vi "Dash Read.vi"(0 "Auto Options":T5={"Starting Position"=enum."Left L1 ", "First Score Pos"=enum."7", "Second Score Pos"=enum."5"}, 2 "PID gains A":T1={"proportional gain (Kc)"=0.039, "integral time (Ti, min)"=0.0, "derivative time (Td, min)"=0.0018000000000000004} {"derivative time (Td, min)" format="%.4f"; "integral time (Ti, min)" format="%.4f"; "proportional gain (Kc)" format="%.4f"}, 3 "PID gains B":T1={"proportional gain (Kc)"=0.027999999999999997, "integral time (Ti, min)"=0.0, "derivative time (Td, min)"=0.0018000000000000004} {"derivative time (Td, min)" format="%.4f"; "integral time (Ti, min)" format="%.4f"; "proportional gain (Kc)" format="%.4f"}) -> (12 "Competion":string, 14 "Replay Number":dbl, 15 "Match Number":dbl, 16 "Match Type":string, 17 "output cluster":T2, 18 "Pressure":dbl, 19 "AutoValid?":bool)   [LabVIEW 2018]
uses:
  Subsystems/Drive/MotionProfile/StartingPosition.ctl
  Subsystems/Drive/MotionProfile/Path_Decider.ctl
  <vilib>/Rock Robotics/Network Tables/NT Read Boolean.vi
  <vilib>/Rock Robotics/Network Tables/NT Write Variant.vi
  <vilib>/Rock Robotics/Network Tables/NT Read Number.vi
  <vilib>/Rock Robotics/Network Tables/NT Read String.vi
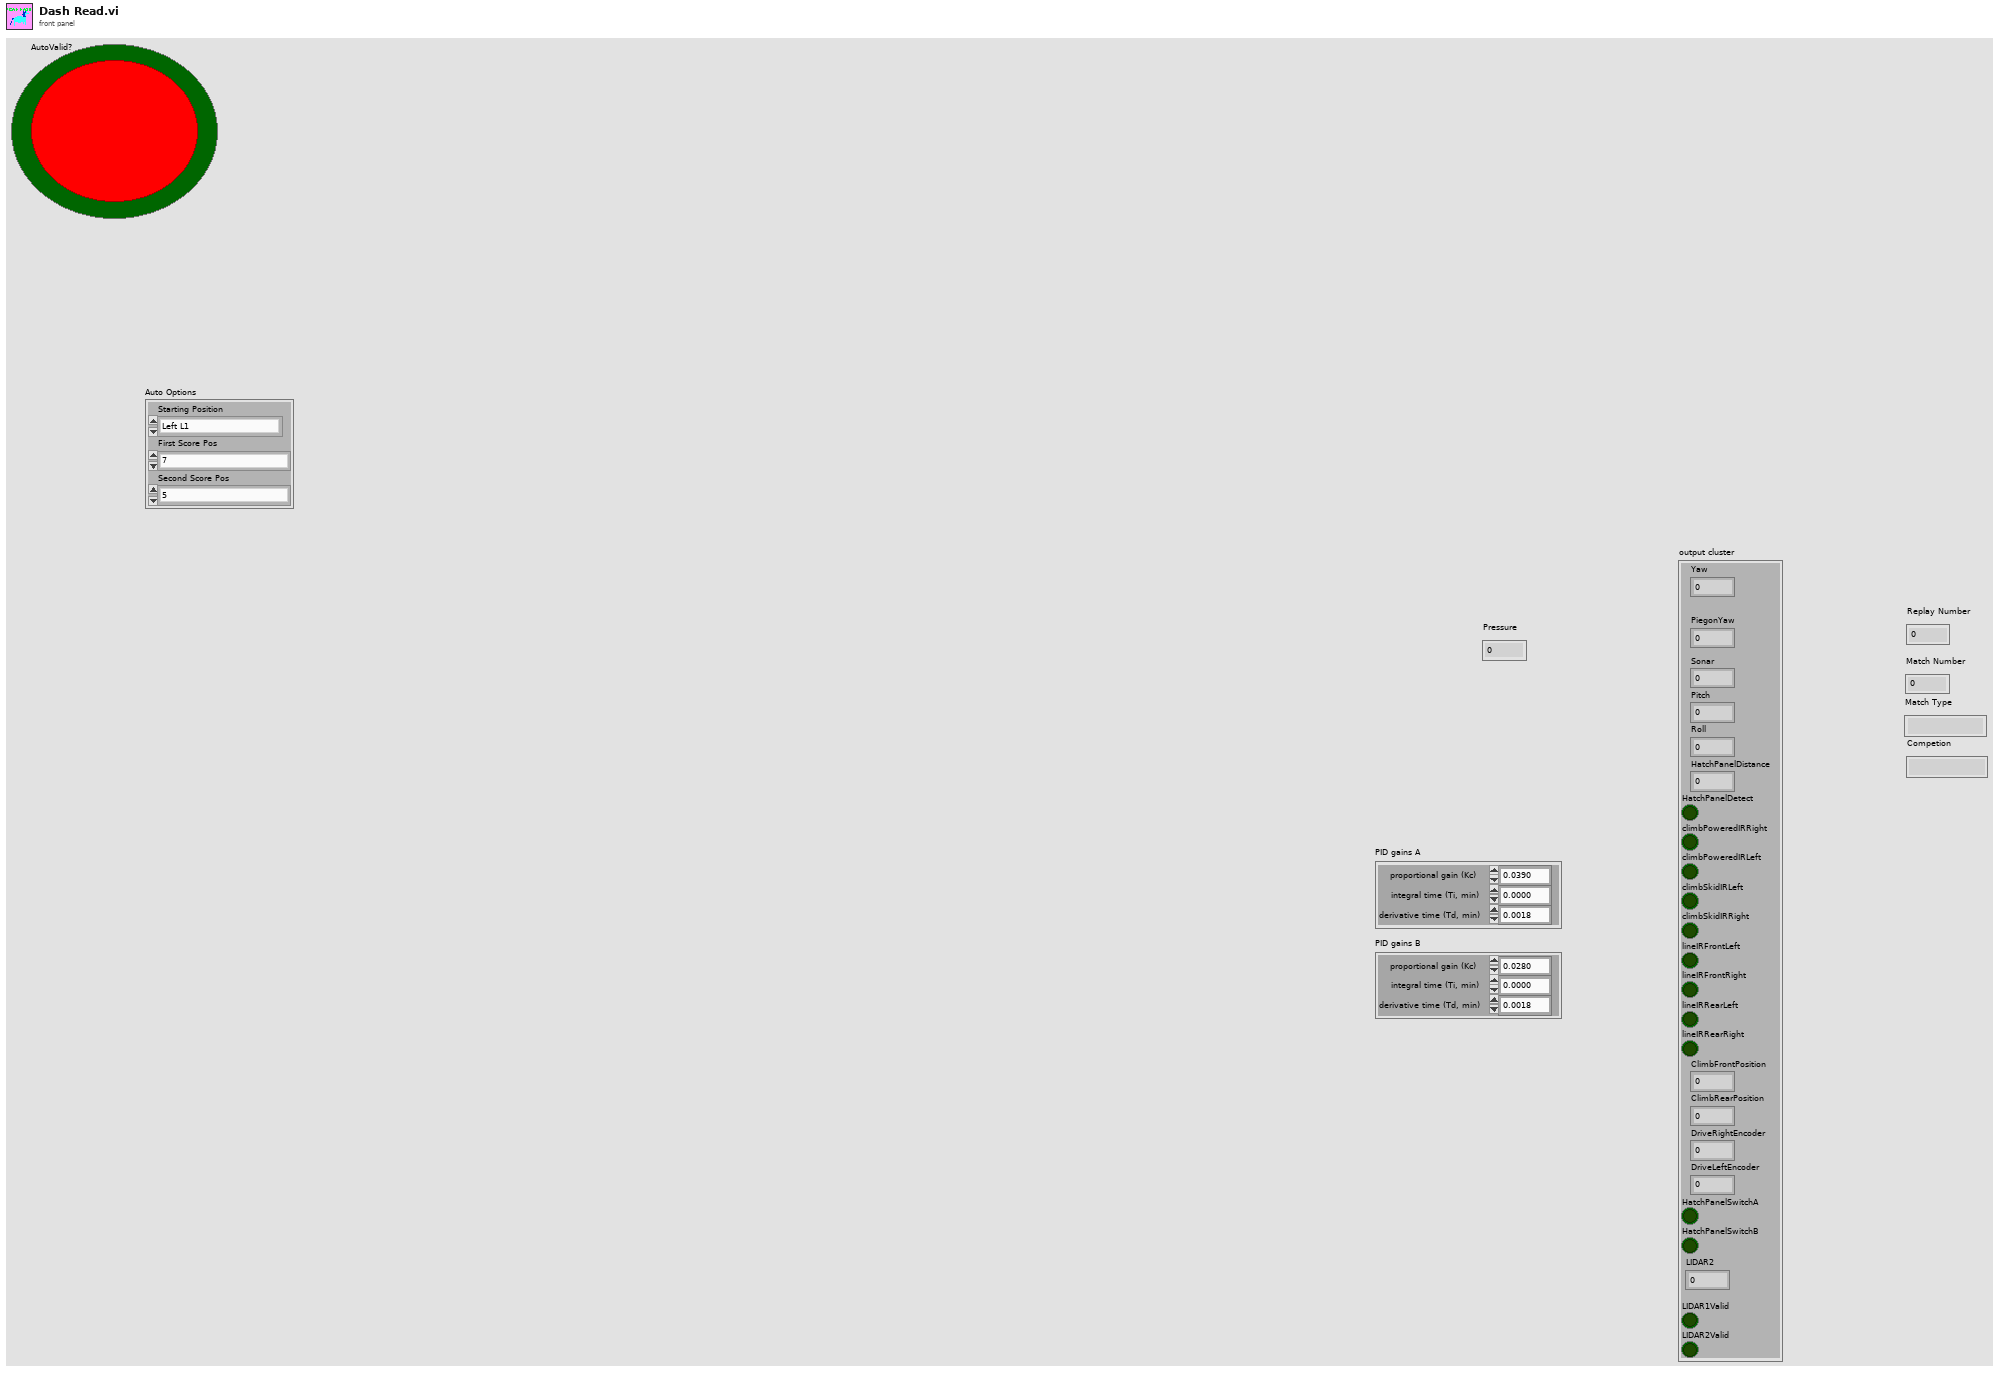
[diagram p1: front panel]
types:
  T1 = cluster{"proportional gain (Kc)":dbl, "integral time (Ti, min)":dbl, "derivative time (Td, min)":dbl}
  T2 = cluster{"Yaw":dbl, "Sonar":dbl, "Pitch":dbl, "Roll":dbl, "HatchPanelDistance":dbl, "HatchPanelDetect":bool, "climbPoweredIRRight":bool, "climbPoweredIRLeft":bool, "climbSkidIRLeft":bool, "climbSkidIRRight":bool, "lineIRFrontLeft":bool, "lineIRFrontRight":bool, "lineIRRearLeft":bool, "lineIRRearRight":bool, "ClimbFrontPosition":dbl, "ClimbRearPosition":dbl, "DriveRightEncoder":dbl, "DriveLeftEncoder":dbl, "HatchPanelSwitchA":bool, "HatchPanelSwitchB":bool, "LIDAR2":dbl, "PiegonYaw":dbl, "LIDAR2Valid":bool, "LIDAR1Valid":bool}
  T3 = typedef "StartingPosition.ctl" = enum16{"Left L1 ", "Middle L1", "Right L1", "Left L2", "Right L2", "Don't Move"}
  T4 = typedef "Path_Decider.ctl" = enum16{"1", "2", "3", "4", "5", "6", "7", "8", "Left_Rocket_Front", "Left_Rocket_Rear", "Right_Rocket_Front", "Right_Rocket_Rear"}
  T5 = cluster{"Starting Position":T3, "First Score Pos":T4, "Second Score Pos":T4}
  T6 = cluster{"Yaw":dbl, "Sonar":dbl, "Pitch":dbl, "Roll":dbl, "HatchPanelDistance":dbl, "HatchPanelDetect":bool, "climbPoweredIRRight":bool, "climbPoweredIRLeft":bool, "climbSkidIRLeft":bool, "climbSkidIRRight":bool, "lineIRFrontLeft":bool, "lineIRFrontRight":bool, "lineIRRearLeft":bool, "lineIRRearRight":bool, "ClimbFrontPosition":dbl, "ClimbRearPosition":dbl, "DriveRightEncoder":dbl, "DriveLeftEncoder":dbl, "HatchPanelSwitchA":bool, "HatchPanelSwitchB":bool, "LIDAR2":dbl, "PigeonYaw":dbl, "LIDAR1Valid":bool, "LIDAR2Valid":bool}
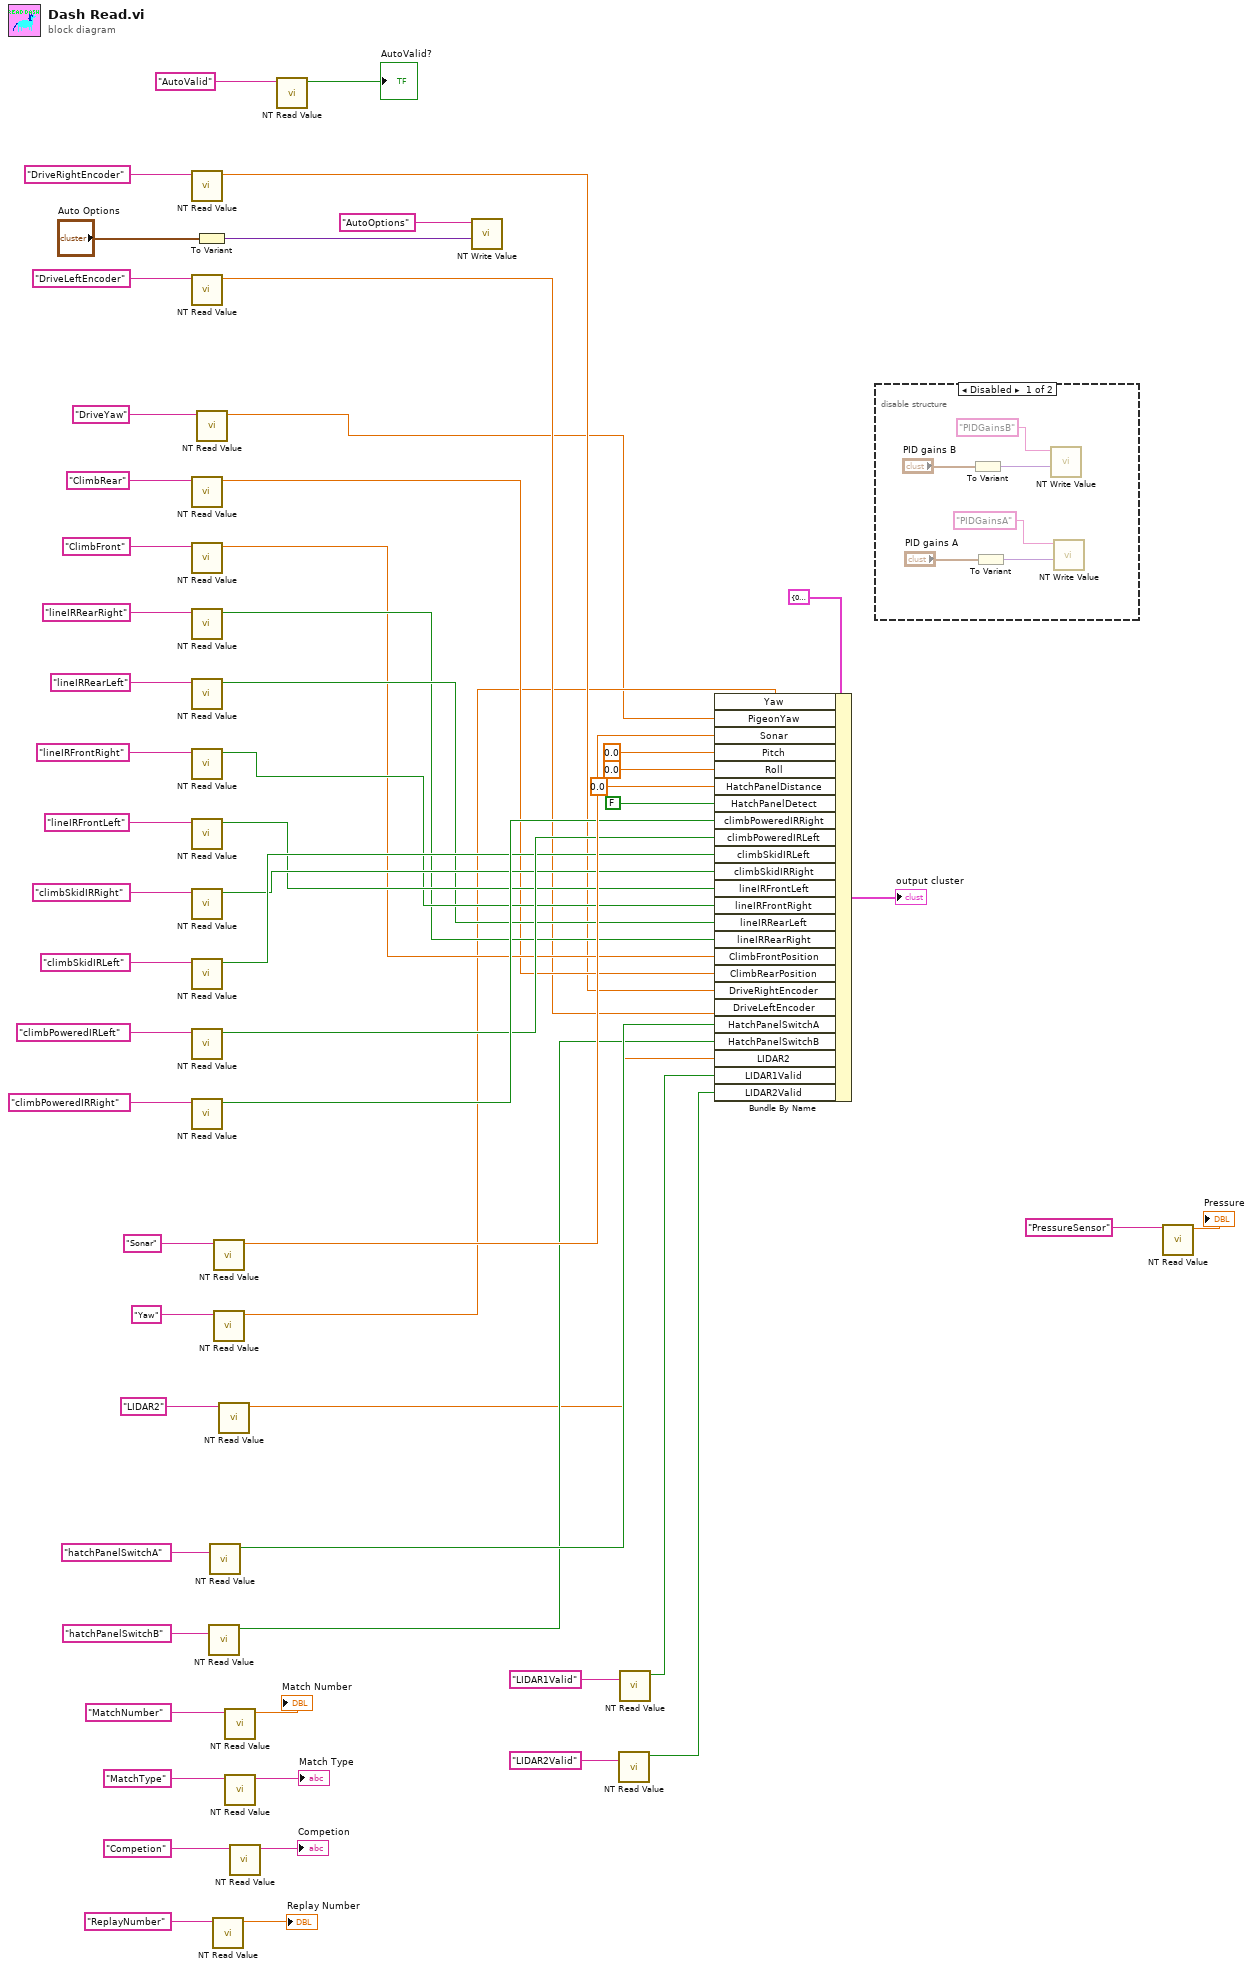
[diagram p0: block diagram]
diagram:
  n1 = call-poly <vilib>:"NT Read Value.vi"("Name"="DriveRightEncoder") -> ("Numeric"=w30:dbl)  [unwired: 9 in, 1 out]
  n2 = call-poly <vilib>:"NT Read Value.vi"("Name"="DriveLeftEncoder") -> ("Numeric"=w29:dbl)  [unwired: 9 in, 1 out]
  n3 = call-poly <vilib>:"NT Read Value.vi"("Name"="ClimbRear") -> ("Numeric"=w31:dbl)  [unwired: 9 in, 1 out]
  n4 = call-poly <vilib>:"NT Read Value.vi"("Name"="ClimbFront") -> ("Numeric"=w32:dbl)  [unwired: 9 in, 1 out]
  n5 = call-poly <vilib>:"NT Read Value.vi"("Name"="lineIRRearRight") -> ("Boolean"=w33:bool)  [unwired: 9 in, 1 out]
  n6 = call-poly <vilib>:"NT Read Value.vi"("Name"="lineIRRearLeft") -> ("Boolean"=w34:bool)  [unwired: 9 in, 1 out]
  n7 = call-poly <vilib>:"NT Read Value.vi"("Name"="lineIRFrontRight") -> ("Boolean"=w35:bool)  [unwired: 9 in, 1 out]
  n8 = call-poly <vilib>:"NT Read Value.vi"("Name"="lineIRFrontLeft") -> ("Boolean"=w36:bool)  [unwired: 9 in, 1 out]
  n9 = call-poly <vilib>:"NT Read Value.vi"("Name"="climbSkidIRRight") -> ("Boolean"=w37:bool)  [unwired: 9 in, 1 out]
  n10 = call-poly <vilib>:"NT Read Value.vi"("Name"="climbSkidIRLeft") -> ("Boolean"=w38:bool)  [unwired: 9 in, 1 out]
  n11 = call-poly <vilib>:"NT Read Value.vi"("Name"="climbPoweredIRLeft") -> ("Boolean"=w39:bool)  [unwired: 9 in, 1 out]
  n12 = call-poly <vilib>:"NT Read Value.vi"("Name"="climbPoweredIRRight") -> ("Boolean"=w40:bool)  [unwired: 9 in, 1 out]
  n13 = To Variant(anything="Auto Options") -> (Variant=w51:variant)
  n14 = call-poly <vilib>:"NT Read Value.vi"("Name"="DriveYaw") -> ("Numeric"=w7:dbl)  [unwired: 9 in, 1 out]
  n15 = call-poly <vilib>:"NT Read Value.vi"("Name"="hatchPanelSwitchB") -> ("Boolean"=w25:bool)  [unwired: 9 in, 1 out]
  n16 = call-poly <vilib>:"NT Read Value.vi"("Name"="hatchPanelSwitchA") -> ("Boolean"=w26:bool)  [unwired: 9 in, 1 out]
  n17 = call-poly <vilib>:"NT Read Value.vi"("Name"="ReplayNumber") -> ("Numeric"=→"Replay Number":dbl)  [unwired: 9 in, 1 out]
  n18 = call-poly <vilib>:"NT Read Value.vi"("Name"="Sonar") -> ("Numeric"=w41:dbl)  [unwired: 9 in, 1 out]
  n19 = call-poly <vilib>:"NT Read Value.vi"("Name"="Yaw") -> ("Numeric"=w13:dbl)  [unwired: 9 in, 1 out]
  n20 = call-poly <vilib>:"NT Read Value.vi"("Name"="LIDAR2") -> ("Numeric"=w8:dbl)  [unwired: 9 in, 1 out]
  n21 = call-poly <vilib>:"NT Read Value.vi"("Name"="MatchNumber") -> ("Numeric"=→"Match Number":dbl)  [unwired: 9 in, 1 out]
  n22 = call-poly <vilib>:"NT Read Value.vi"("Name"="MatchType") -> ("String"=→"Match Type":string)  [unwired: 9 in, 1 out]
  n23 = call-poly <vilib>:"NT Read Value.vi"("Name"="Competion") -> ("String"=→"Competion":string)  [unwired: 9 in, 1 out]
  n24 = call-poly <vilib>:"NT Read Value.vi"("Name"="AutoValid") -> ("Boolean"=→"AutoValid?":bool)  [unwired: 9 in, 1 out]
  n25 = call-poly <vilib>:"NT Write Value.vi"("Variant"=w51, "Name"="AutoOptions") -> ()  [unwired: 9 in, 1 out]
  n26 = call-poly <vilib>:"NT Read Value.vi"("Name"="LIDAR2Valid") -> ("Boolean"=w3:bool)  [unwired: 9 in, 1 out]
  n27 = call-poly <vilib>:"NT Read Value.vi"("Name"="LIDAR1Valid") -> ("Boolean"=w4:bool)  [unwired: 9 in, 1 out]
  n28 = Bundle By Name(cluster=T6 {"Yaw"=0.0, "Sonar"=0.0, "Pitch"=0.0, "Roll"=0.0, "HatchPanelDistance"=0.0, "HatchPanelDetect"=FALSE, "climbPoweredIRRight"=FALSE, "climbPoweredIRLeft"=FALSE, "climbSkidIRLeft"=FALSE, "climbSkidIRRight"=FALSE, "lineIRFrontLeft"=FALSE, "lineIRFrontRight"=FALSE, "lineIRRearLeft"=FALSE, "lineIRRearRight"=FALSE, "ClimbFrontPosition"=0.0, "ClimbRearPosition"=0.0, "DriveRightEncoder"=0.0, "DriveLeftEncoder"=0.0, "HatchPanelSwitchA"=FALSE, "HatchPanelSwitchB"=FALSE, "LIDAR2"=0.0, "PigeonYaw"=0.0, "LIDAR1Valid"=FALSE, "LIDAR2Valid"=FALSE} ("Important Robot Data"), "Yaw"=w13, "PigeonYaw"=w7, "Sonar"=w41, "Pitch"=0.0, "Roll"=0.0, "HatchPanelDistance"=0.0, "HatchPanelDetect"=FALSE, "climbPoweredIRRight"=w40, "climbPoweredIRLeft"=w39, "climbSkidIRLeft"=w38, "climbSkidIRRight"=w37, "lineIRFrontLeft"=w36, "lineIRFrontRight"=w35, "lineIRRearLeft"=w34, "lineIRRearRight"=w33, "ClimbFrontPosition"=w32, "ClimbRearPosition"=w31, "DriveRightEncoder"=w30, "DriveLeftEncoder"=w29, "HatchPanelSwitchA"=w26, "HatchPanelSwitchB"=w25, "LIDAR2"=w8, "LIDAR1Valid"=w4, "LIDAR2Valid"=w3) -> (→"output cluster":T6)
  n29 = disable-structure shown="Disabled" {
    frame Disabled {
      n30 = To Variant(anything="PID gains B") -> (Variant=w63:variant)
      n31 = To Variant(anything="PID gains A") -> (Variant=w65:variant)
      n32 = call-poly <vilib>:"NT Write Value.vi"("Variant"=w63, "Name"="PIDGainsB") -> ()  [unwired: 9 in, 1 out]
      n33 = call-poly <vilib>:"NT Write Value.vi"("Variant"=w65, "Name"="PIDGainsA") -> ()  [unwired: 9 in, 1 out]
    }
    frame Enabled {
    }
  }
  n34 = call-poly <vilib>:"NT Read Value.vi"("Name"="PressureSensor" ("refnum name")) -> ("Numeric"=→"Pressure":dbl)  [unwired: 9 in, 1 out]
